vi "Global_ACT Write_Data Out.vi"() -> ()   [LabVIEW 2017, in "Arm.lvlib"]
uses:
  Arm.lvlib
  CLUSTER_ACT_Lift Output.ctl
  _SHARE ALL/RoboRio Share All/SRX Share All/TypeDefs SRX/Cluster_SRX_Common Runtime Data.ctl
  _SHARE ALL/RoboRio Share All/SRX Share All/TypeDefs SRX/Cluster_SRX_Error Calculations.ctl
  _SHARE ALL/RoboRio Share All/SRX Share All/TypeDefs SRX/Cluster_SRX_Voltage Out Data.ctl
  _SHARE ALL/RoboRio Share All/SRX Share All/TypeDefs SRX/Cluster_SRX_Sensor Out Data.ctl
  _SHARE ALL/RoboRio Share All/SRX Share All/TypeDefs SRX/Cluster_SRX_F and R Limit Indicators.ctl
panel:
  in  "Arm_ACT_Output":T1 {"Common Runtime Data"."Temp" format="%.1f"; "Common Runtime Data"."Voltage"."Bus" format="%.3f"; "Common Runtime Data"."Voltage"."Output" format="%.3f"; "Common Runtime Data"."Voltage"."Percent" format="%.3f"; "Common Runtime Data"."Current" format="%.2f"}
  # "The Names of the Data items in the Global Variable MUST describe who the Single Writer is\nNaming Convention of all Data Items is:   \nLib Name_Loop Name (SM or SEN or ACT)_Data Name\nExamples:\nDrive_ACT_X axis\nGameController_SEN_JoystickLeft\nHopper_SM_AgitatorSpeed"
  # "C"
  # "Units"
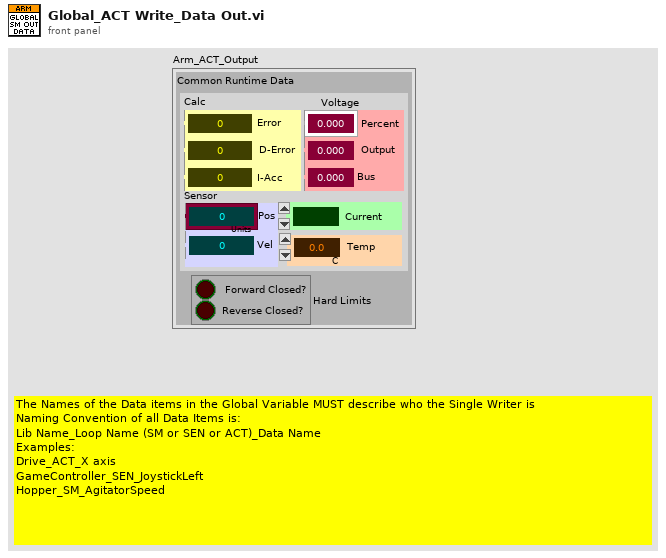
[diagram p1: front panel]
types:
  T1 = typedef "Arm.lvlib/CLUSTER_ACT_Lift Output.ctl" = cluster{"Common Runtime Data":T2, "Hard Limits":T6}
  T2 = typedef "Cluster_SRX_Common Runtime Data.ctl" = cluster{"Calc":T3, "Voltage ":T4, "Sensor":T5, "Current":dbl, "Temp":dbl}
  T3 = typedef "Cluster_SRX_Error Calculations.ctl" = cluster{"Error":i32, "D-Error":dbl, "I-Acc":dbl}
  T4 = typedef "Cluster_SRX_Voltage Out Data.ctl" = cluster{"Percent":dbl, "Output":dbl, "Bus":dbl}
  T5 = typedef "Cluster_SRX_Sensor Out Data.ctl" = cluster{"Pos":i32, "Vel":i32}
  T6 = typedef "Cluster_SRX_F and R Limit Indicators.ctl" = cluster{"Forward Closed?":bool, "Reverse Closed?":bool}
diagram:
